vi "Create Mask By Alpha.vi"(10 "Transparency Thresh":u8=127, 11 "image data":T1) -> (3 "masked image data":T1)   [LabVIEW 2016]
uses:
  imagedata.ctl
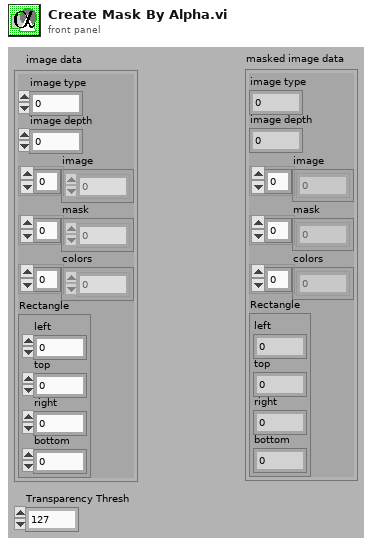
[diagram p1: front panel]
types:
  T1 = typedef "imagedata.ctl" = cluster{"image type":i32, "image depth":i32, "image":u8[], "mask":u8[], "colors":u32[], "Rectangle":cluster{"left":i16, "top":i16, "right":i16, "bottom":i16}}
  T2 = cluster{"left":i16, "top":i16, "right":i16, "bottom":i16}
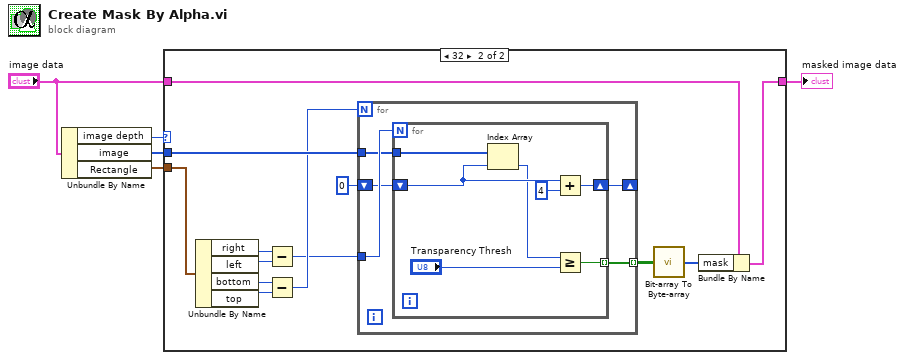
[diagram p0: block diagram]
diagram:
  n1 = Unbundle By Name("image data") -> ("image depth"=w5:i32, "image"=w3:u8[], "Rectangle"=w4:T2)
  n2 = case shown="32" w5 {
    tunnel: w4 -> [_ w19]
    tunnel: w3 -> [_ w14]
    tunnel: "image data" -> [w6 w10]
    tunnel: [w6 w9] -> w1
    frame Default {
    }
    frame 32 {
      n3 = Unbundle By Name(w19) -> ("right"=w18:i16, "left"=w17:i16, "bottom"=w16:i16, "top"=w15:i16)
      n4 = Subtract(x=w18, y=w17) -> (x-y=w7:i16)
      n5 = Subtract(x=w16, y=w15) -> (x-y=w8:i16)
      n6 = for {
        N: w8 -> [_]
        tunnel: w7 -> [w24]
        tunnel: w14 -> [w23]
        shift-right: [w21] -> _
        shift-left: 0 -> [w22]
        tunnel: [w20] -> w12 mode=indexing
        n7 = for {
          N: w24 -> [_]
          tunnel: w23 -> [w31]
          shift-right: [w30] -> w21
          shift-left: w22 -> [w29]
          tunnel: [w25] -> w20 mode=indexing
          n8 = Index Array(array=w31, index=w29) -> (element=w27:u8)
          n9 = Add(x=w29, y=4) -> (x+y=w30:i32)
          n10 = Greater Or Equal?(x=w27, y="Transparency Thresh") -> (x >= y?=w25:bool)
        }
      }
      n11 = call "Bit-array To Byte-array.vi"("bit array"=w12) -> ("byte array"=w11:u8[])
      n12 = Bundle By Name(cluster=w10, "mask"=w11) -> (w9:T1)
    }
  }
  "masked image data" <- w1
